vi "Player Reset.vi"(8 "error in (no error)":errorcluster, 10 "Starting Coordinate":T1, 11 "Player in":refnum<class "Player.lvclass">) -> (0 "error out":errorcluster, 3 "Player out":refnum<class "Player.lvclass">)   [LabVIEW 2019, in "Player.lvclass"]
uses:
  Player.lvclass
  Snake/Snake.lvclass
  Coordinate STYP.ctl
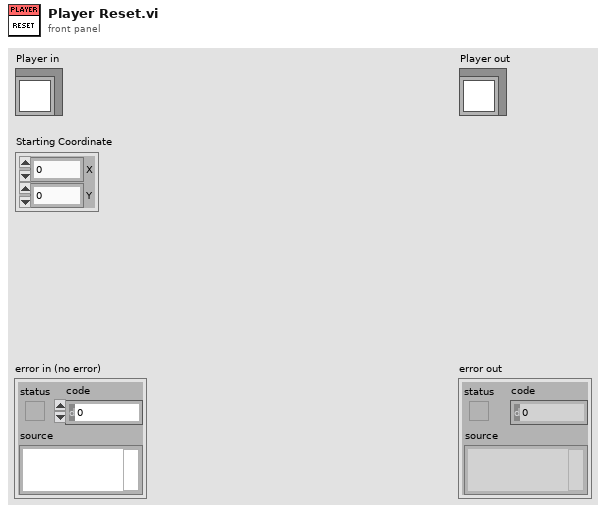
[diagram p1: front panel]
types:
  T1 = typedef "Coordinate STYP.ctl" = cluster{"X":i32, "Y":i32}
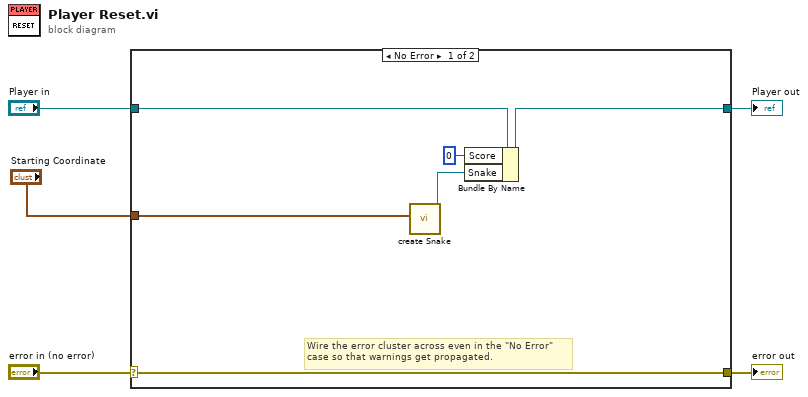
[diagram p0: block diagram]
diagram:
  n1 = case shown="No Error" "error in (no error)" {
    selector: "error in (no error)" -> [w11 w13]
    tunnel: [w11 w13] -> w4
    tunnel: [w10 w12] -> w2
    tunnel: "Player in" -> [w9 w12]
    tunnel: "Starting Coordinate" -> [w7 _]
    frame No Error {
      # "Wire the error cluster across even in the \"No Error\"\ncase so that warnings get propagated."
      n2 = call "create Snake.vi"("Coordinate"=w7) -> ("Snake out"=w8:refnum<class "Snake.lvclass">)  [unwired: 9 in, 1 out]
      n3 = Bundle By Name(cluster=w9, "Score"=u32 0, "Snake"=w8) -> (w10:refnum<class "Player.lvclass">)
    }
    frame Error {
    }
  }
  "error out" <- w4
  "Player out" <- w2
